vi "AIDI-Create Channels (AI).vi"(0 "Tasks In":T1[](array[typedef]), 7 "Fs (Hz)":dbl, 9 "Npts":i32, 11 "error in (no error)":errorcluster) -> (4 "Tasks Out":T1[](array[typedef]), 15 "error out":errorcluster)   [LabVIEW 2020]
uses:
  Typedefs/AIDI-Task Specification.ctl
  <vilib>/DAQmx/create/channels.llb/DAQmx Create Channel (AI-Voltage-Basic).vi
  <vilib>/DAQmx/configure/timing.llb/DAQmx Timing (Sample Clock).vi
  <resource>/objmgr/daqmx.rc
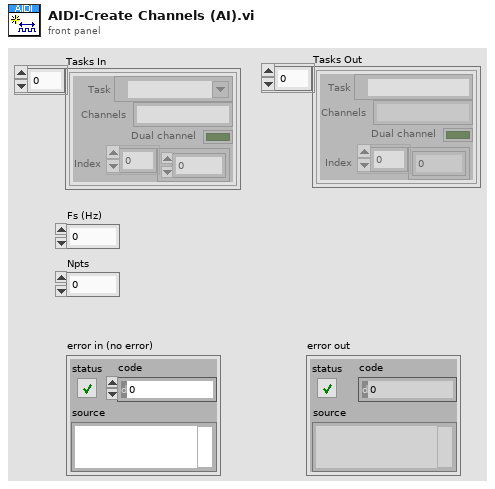
[diagram p1: front panel]
types:
  T1 = typedef "AIDI-Task Specification.ctl" = cluster{"Task":refnum<k21>, "Channels":string, "Dual channel":bool, "Index":i32[]}
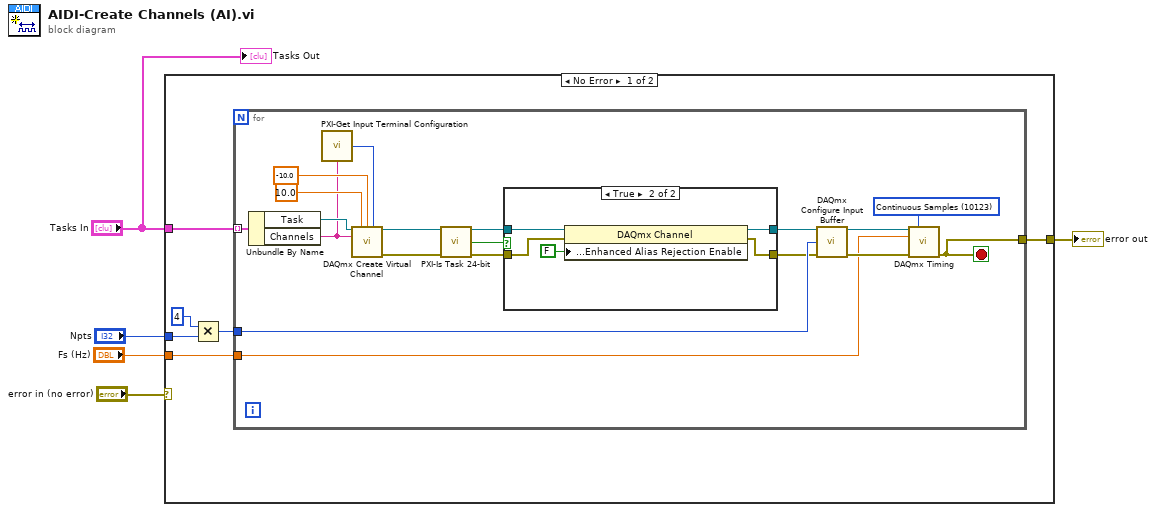
[diagram p0: block diagram]
diagram:
  n1 = case shown="No Error" "error in (no error)" {
    selector: "error in (no error)" -> [_ w38]
    tunnel: "Tasks In" -> [w11 _]
    tunnel: "Fs (Hz)" -> [w10 _]
    tunnel: "Npts" -> [w8 _]
    tunnel: [w6 w38] -> w2
    frame No Error {
      n2 = Multiply(x=4 ("y"), y=w8) -> (x*y=w7:i32)
      n3 = for {
        tunnel: w11 -> [w30] mode=indexing
        tunnel: w7 -> [w21]
        tunnel: w10 -> [w24]
        tunnel: [w28] -> w6
        stop <- w28 stop-if-true
        w25 = 10123 items=["Finite Samples"=10178, "Continuous Samples"=10123, "Hardware Timed Single Point"=12522] ("sample mode")
        n4 = Unbundle By Name(w30) -> ("Task"=w29:refnum<k21>, "Channels"=w13:string)
        n5 = call "PXI-Get Input Terminal Configuration.vi"("channel"=w13) -> ("term config out"=w12:i32)  [unwired: 13 in, 1 out]
        n6 = call-poly <vilib>:"DAQmx Create Virtual Channel.vi"("task in"=w29, "maximum value"=10.0, "minimum value"=-10.0, "input terminal configuration"=w12, "physical channels"=w13) -> ("task out"=w22:refnum<k21>, "error out"=w23:errorcluster)  [unwired: 9 in]
        n7 = call "PXI-Is Task 24-bit.vi"("task"=w22, "error in (no error)"=w23) -> ("task out"=w19:refnum<k21>, "is 24bit?"=w20:bool, "error out"=w18:errorcluster)  [unwired: 8 in, 3 out]
        n8 = case shown="True" w20 {
          tunnel: w19 -> [w32 w37]
          tunnel: w18 -> [w31 w36]
          tunnel: [w31 w34] -> w17
          tunnel: [w32 w33] -> w16
          frame False {
          }
          frame True {
            n9 = property class="DAQmx Channel"(reference=w37, error in=w36, "Analog Input:General Properties:Advanced:Enhanced Alias Rejection Enable"=FALSE ("AI.EnhancedAliasRejectionEnable")) -> (reference out=w33:refnum<k21>, error out=w34:errorcluster)
          }
        }
        n10 = call <vilib>:"DAQmx Configure Input Buffer.vi"("task/channels in"=w16, "buffer size (in samples per channel)"=w21, "error in"=w17) -> ("task out"=w27:refnum<k21>, "error out"=w26:errorcluster)  [unwired: 11 in]
        n11 = call-poly <vilib>:"DAQmx Timing.vi"("task/channels in"=w27, "sample mode"=w25, "rate"=w24, "error in"=w26) -> ("error out"=w28:errorcluster)  [unwired: 10 in, 1 out]
      }
    }
    frame Error {
    }
  }
  "error out" <- w2
  "Tasks Out" <- "Tasks In"
